vi "PH_4_Pos_Selector.PC set Position.vi"(0 "i ref in":refnum<vi>, 2 "Wanted Position":T1 items=["unknown", "Position I", "Position II", "Position III", "Position IV", "moving"], 5 "error IO":errorcluster) -> (14 "i ref out":refnum<vi>, 19 "error out":errorcluster)   [LabVIEW 2014, in "PH_4_Pos_Selector.lvlib"]
uses:
  PH_4_Pos_Selector.lvlib
  PH_4_Pos_Selector.Position Selector.ctl
  PH_Basics/PH_AxisGUI_BaseClass/PH_AxisGUI_BaseClass.lvlib
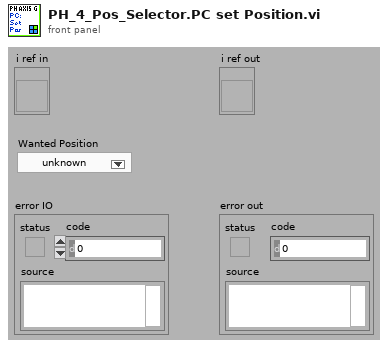
[diagram p1: front panel]
types:
  T1 = typedef "PH_4_Pos_Selector.lvlib/PH_4_Pos_Selector.Position Selector.ctl" = u16
  T2 = typedef "PH_4_Pos_Selector.lvlib/PH_4_Pos_Selector.i attribute.ctl" = cluster{"GUI Refs":cluster{"Position I":refnum<vi>, "Position II":refnum<vi>, "Position III":refnum<vi>, "Position IV":refnum<vi>, "rel. Mode?":refnum<vi>, "Define Selector":refnum<vi>}, "Current Position":T1, "Service ID Position":i32, "Position Array":T3[], "Description Array":string[], "relative Mode":bool, "Wanted Define Selector Position":string}
  T3 = typedef "PH_4_Pos_Selector.lvlib/PH_4_Pos_Selector.Position.ctl" = cluster{"Axis 1":dbl, "Axis 2":dbl}
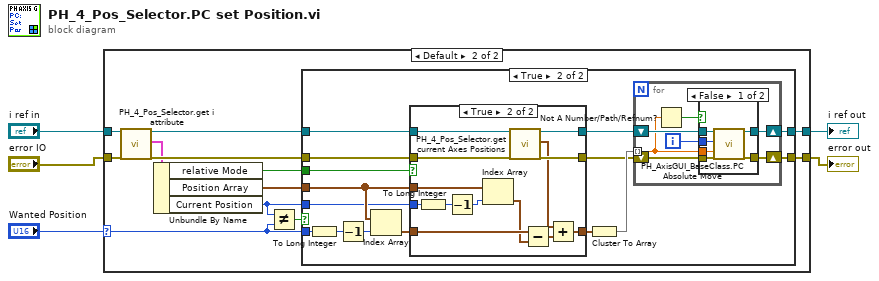
[diagram p0: block diagram]
diagram:
  n1 = case shown="Default" "Wanted Position" {
    selector: "Wanted Position" -> [_ w11]
    tunnel: "i ref in" -> [w7 w19]
    tunnel: "error IO" -> [w6 w18]
    tunnel: [w7 w13] -> w3
    tunnel: [w6 w15] -> w4
    frame 0 {
    }
    frame Default {
      n2 = call "PH_4_Pos_Selector.get i attribute.vi"("i ref in"=w19, "error in (no error)"=w18) -> ("i ref out"=w14:refnum<vi>, "i attribute"=w16:T2, "error out"=w17:errorcluster)  [unwired: 15 in]
      n3 = Unbundle By Name(w16) -> ("relative Mode"=w9:bool, "Position Array"=w10:T3[], "Current Position"=w8:T1)
      n4 = Not Equal?(x=w8, y=w11) -> (x != y?=w12:bool)
      n5 = case shown="True" w12 {
        tunnel: w17 -> [w20 w26]
        tunnel: [w20 w36] -> w15
        tunnel: w14 -> [w21 w27]
        tunnel: [w21 w35] -> w13
        tunnel: w11 -> [_ w33]
        tunnel: w10 -> [_ w23]
        tunnel: w9 -> [_ w30]
        tunnel: w8 -> [_ w22]
        frame False {
        }
        frame True {
          n6 = To Long Integer(number=w33) -> (32bit integer=w32:i32)
          n7 = Decrement(x=w32) -> (x-1=w31:i32)
          n8 = Index Array(array=w23, index=w31) -> (element=w29:T3)
          n9 = case shown="True" w30 {
            tunnel: w29 -> [w39 w44]
            tunnel: [w39 w40] -> w28
            tunnel: w27 -> [w38 w52]
            tunnel: w26 -> [w37 w51]
            tunnel: [w38 w50] -> w25
            tunnel: [w37 w49] -> w24
            tunnel: w23 -> [_ w46]
            tunnel: w22 -> [_ w45]
            frame False {
            }
            frame True {
              n10 = To Long Integer(number=w45) -> (32bit integer=w48:i32)
              n11 = Decrement(x=w48) -> (x-1=w47:i32)
              n12 = Index Array(array=w46, index=w47) -> (element=w43:T3)
              n13 = call "PH_4_Pos_Selector.get current Axes Positions.vi"("VI in"=w52, "error in (no error)"=w51) -> ("VI out"=w50:refnum<vi>, "Current Axes Positions"=w42:T3, "error out"=w49:errorcluster)  [unwired: 13 in, 2 out]
              n14 = Subtract(x=w44, y=w43) -> (x-y=w41:T3)
              n15 = Add(x=w42, y=w41) -> (x+y=w40:T3)
            }
          }
          n16 = Cluster To Array(cluster=w28) -> (array=w34:dbl[])
          n17 = for {
            tunnel: w34 -> [w55] mode=indexing
            shift-right: [w56] -> w35
            shift-left: w25 -> [w57]
            shift-right: [w58] -> w36
            shift-left: w24 -> [w59]
            i -> [w54]
            n18 = Not A Number/Path/Refnum?(number/path/refnum=w55) -> (NaN/Path/Refnum?=w53:bool)
            n19 = case shown="False" w53 {
              tunnel: w59 -> [w65 w66]
              tunnel: [w64 w66] -> w58
              tunnel: w57 -> [w63 w67]
              tunnel: [w62 w67] -> w56
              tunnel: w55 -> [w61 _]
              tunnel: w54 -> [w60 _]
              frame False {
                n20 = call "PH_AxisGUI_BaseClass.PC Absolute Move.vi"("i ref in"=w63, "Axis"=w60, "Position [Units]"=w61, "error in"=w65) -> ("i ref out"=w62:refnum<vi>, "error out"=w64:errorcluster)  [unwired: 14 in]
              }
              frame True {
              }
            }
          }
        }
      }
    }
  }
  "error out" <- w4
  "i ref out" <- w3
